vi "Send Emailwithout attachment.vi"(0 "To: 2":string="pankaj7897@outlook.com", 1 "Subject 2":string="ghgtr", 2 "Message 2":string="rttwq") -> ()   [LabVIEW 2013]
doc: "Uses the SMTP Email Client to send an email to a standard or secure SMTP server."
uses:
  <vilib>/smtpClient/Set Message Text.vi
  <vilib>/smtpClient/LabVIEWSMTPClient.lvlib
panel:
  in  "Password 2":string="itain'tme"
  in  "Username 2":string="astitva19@hotmail.com"
  in  "Port 2":string="587"
  in  "Sender's Email Address 2":string="astitva19@hotmail.com"
  in  "Outgoing Mail Server (SMTP) 2":string="smtp.live.com"
  # "Outgoing Mail Server"
  # "Optional Parameters"
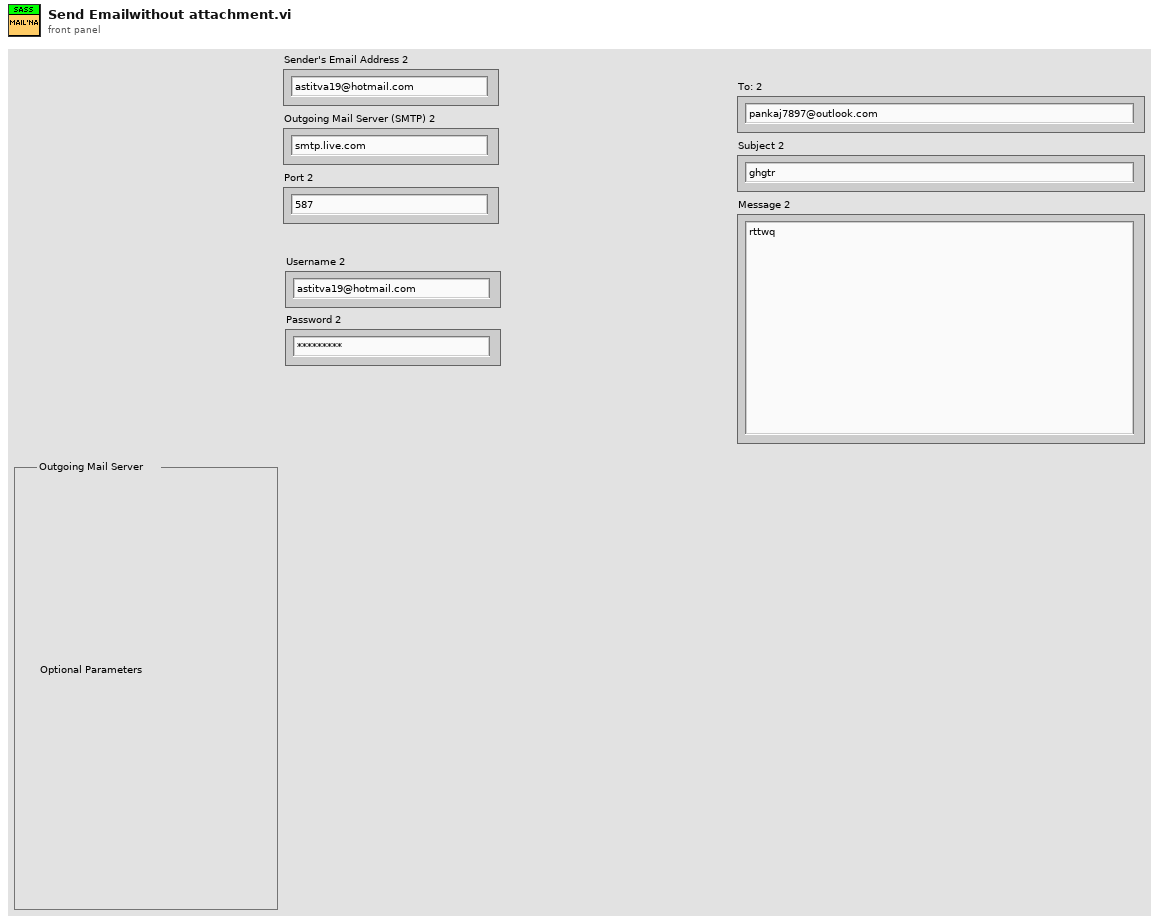
[diagram p1: front panel]
types:
  T1 = typedef "LabVIEWSMTPClient.lvlib/SmtpClientHandle.ctl" = refnum<k1>
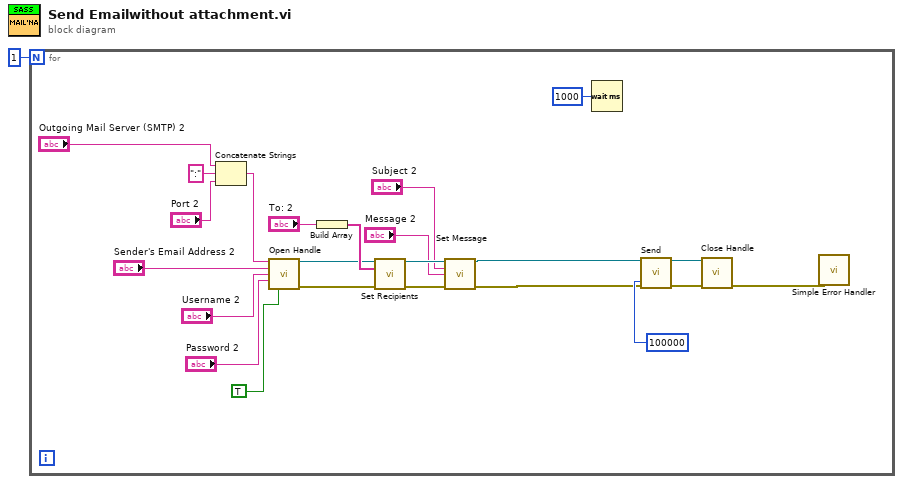
[diagram p0: block diagram]
diagram:
  n1 = for {
    N: 1 -> [_]
    n2 = Concatenate Strings("Outgoing Mail Server (SMTP) 2", ":" ("string"), "Port 2") -> (w21:string)
    n3 = call <vilib>:"Open Handle.vi"("server address"=w21, "from"="Sender's Email Address 2", "username"="Username 2", "password"="Password 2", "use TLS (false)"=TRUE) -> ("handle out"=w10:T1, "error out"=w9:errorcluster)  [unwired: 9 in]
    n4 = Build Array("To: 2") -> (w12:string[])
    n5 = call <vilib>:"Set Recipients.vi"("handle in"=w10, "to"=w12, "error in (no error)"=w9) -> ("handle out"=w16:T1, "error out"=w13:errorcluster)  [unwired: 11 in]
    n6 = call-poly <vilib>:"Set Message.vi"("handle in"=w16, "subject"="Subject 2", "plain text message"="Message 2", "error in (no error)"=w13) -> ("handle out"=w2:T1, "error out"=w3:errorcluster)  [unwired: 10 in]
    n7 = Wait (ms)(milliseconds to wait=u32 1000) -> ()  [unwired: 1 out]
    n8 = call <vilib>:"Send.vi"("handle in"=w2, "error in (no error)"=w3, "timeout in ms (10000)"=100000 ("timeout in ms")) -> ("handle out"=w8:T1, "error out"=w7:errorcluster)  [unwired: 10 in, 1 out]
    n9 = call <vilib>:"Close Handle.vi"("handle in"=w8, "error in (no error)"=w7) -> ("error out"=w5:errorcluster)  [unwired: 12 in, 1 out]
    n10 = call <vilib>:"Simple Error Handler.vi"("error in (no error)"=w5) -> ()  [unwired: 4 in, 5 out]
  }
